vi "Configure Modulation Low Level (PM Function).vi"(8 "error in":errorcluster, 10 "Modulation Waveform (Sine)":T1(ring), 11 "VISA resource name":refnum<visa-resource-name>) -> (0 "error out":errorcluster, 3 "VISA resource name out":refnum<visa-resource-name>)   [LabVIEW 2017, in "Keithley 3390.lvlib"]
doc: "Sets the waveform function of the internal modulating source signal."
uses:
  Keithley 3390.lvlib
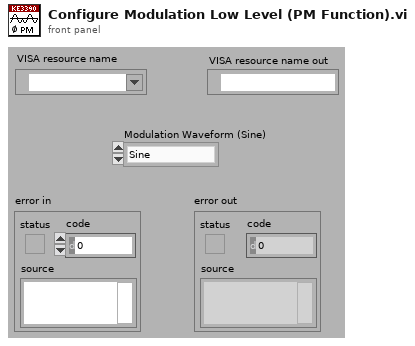
[diagram p1: front panel]
types:
  T1 = enum16{"Sine", "Square", "Ramp", "Negative Ramp", "Triangle", "Noise", "Arbitrary"}
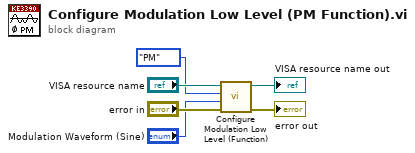
[diagram p0: block diagram]
diagram:
  n1 = call "Configure Modulation Low Level (Function).vi"("error in (no error)"="error in", "Function (Sine)"="Modulation Waveform (Sine)", "Modulation (AM)"=enum16{"AM", "FM", "PM", "PWM"}."PM" ("Modulation (0:AM)"), "VISA resource name"="VISA resource name") -> ("error out"=→"error out":errorcluster, "VISA resource name out"=→"VISA resource name out":refnum<visa-resource-name>)  [unwired: 6 in]
